vi "Write Control Master.vi"(8 "error in (no error)":errorcluster, 10 "Control Master":bool, 11 "Output in":refnum<class "Output.lvclass">) -> (0 "error out":errorcluster, 3 "Output out":refnum<class "Output.lvclass">)   [LabVIEW 2023, in "HAF.lvlib" / "Output.lvclass"]
uses:
  Output.lvclass
  Output.lvclass/Output.ctl
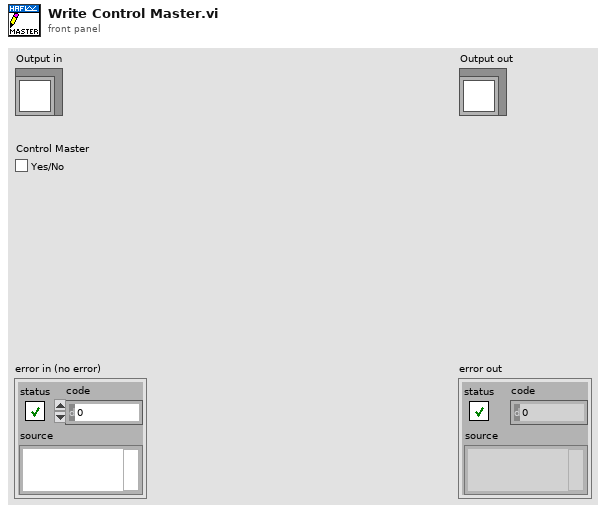
[diagram p1: front panel]
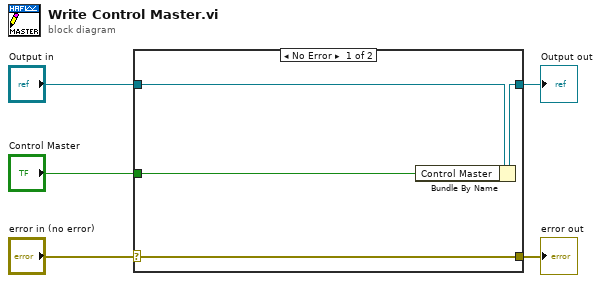
[diagram p0: block diagram]
diagram:
  n1 = case shown="No Error" "error in (no error)" {
    selector: "error in (no error)" -> [w9 w10]
    tunnel: [w9 w10] -> w4
    tunnel: [w7 w11] -> w2
    tunnel: "Output in" -> [w8 w11]
    tunnel: "Control Master" -> [w6 _]
    frame No Error {
      n2 = Bundle By Name(cluster=w8, "Control Master"=w6) -> (w7:refnum<class "Output.lvclass">)
    }
    frame Error {
    }
  }
  "error out" <- w4
  "Output out" <- w2
